vi "Find Devices by Name.vi"(8 "error in":errorcluster, 10 "Device Names":string[](array[string]), 11 "ACNET Devices in":refnum<class "ACNET Devices.lvclass">) -> (0 "error out":errorcluster, 3 "ACNET Devices out":refnum<class "ACNET Devices.lvclass">)   [LabVIEW 2013, in "ACNET Monitor.lvlib"]
uses:
  ACNET Monitor.lvlib
  ACNET Monitor/ACNET Devices.lvclass
  ACNET Monitor/ACNET Device.lvclass
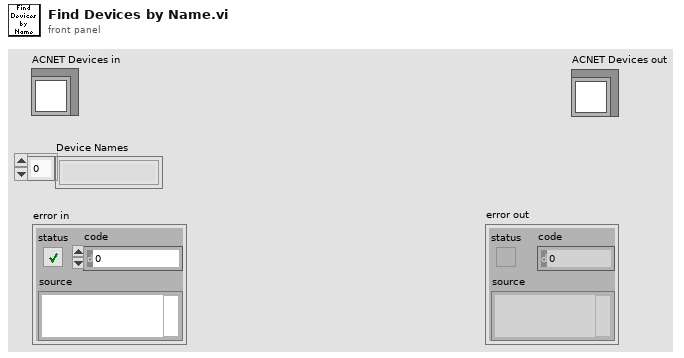
[diagram p1: front panel]
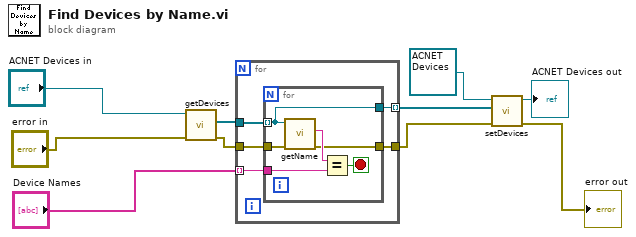
[diagram p0: block diagram]
diagram:
  n1 = call-dynamic "getDevices.vi"("error in (no error)"="error in", "ACNET Devices in"="ACNET Devices in") -> ("error out"=w6:errorcluster, "Devices"=w5:refnum<class "ACNET Device.lvclass">[])  [unwired: 7 in, 1 out]
  n2 = for {
    tunnel: w5 -> [w15]
    tunnel: "Device Names" -> [w13] mode=indexing
    tunnel: w6 -> [w14]
    tunnel: [w12] -> w4 mode=indexing
    tunnel: [w11] -> w10
    n3 = for {
      tunnel: w15 -> [w18] mode=indexing
      tunnel: w14 -> [w21]
      tunnel: w13 -> [w19]
      tunnel: [w18] -> w12
      tunnel: [w16] -> w11
      stop <- w17 stop-if-true
      n4 = call-dynamic "getName.vi"("error in (no error)"=w21, "ACNET Device in"=w18) -> ("error out"=w16:errorcluster, "name"=w20:string)  [unwired: 7 in, 1 out]
      n5 = Equal?(x=w20, y=w19) -> (x = y?=w17:bool)
    }
  }
  n6 = call-dynamic "setDevices.vi"("error in (no error)"=w10, "Devices"=w4, "ACNET Devices in"=refnum<class "ACNET Devices.lvclass"> refnum ("ACNET Devices.lvclass")) -> ("error out"=→"error out":errorcluster, "ACNET Devices out"=→"ACNET Devices out":refnum<class "ACNET Devices.lvclass">)  [unwired: 7 in]
